vi "Get system tasklist.vi"(8 "error in (no error)":errorcluster, 11 "Task to look for":string) -> (0 "error out":errorcluster, 1 "Task found?":bool, 2 "Task count":i32, 3 "Task list":string[](array[string]))   [LabVIEW 2013]
panel:
  out "standard output":string
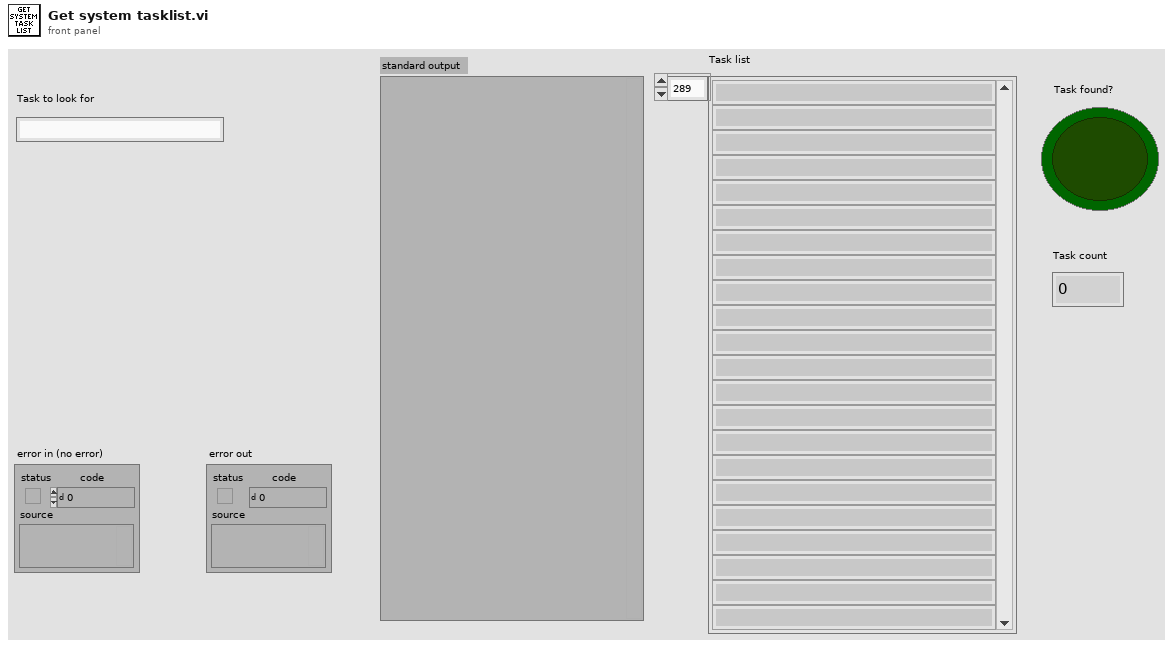
[diagram p1: front panel]
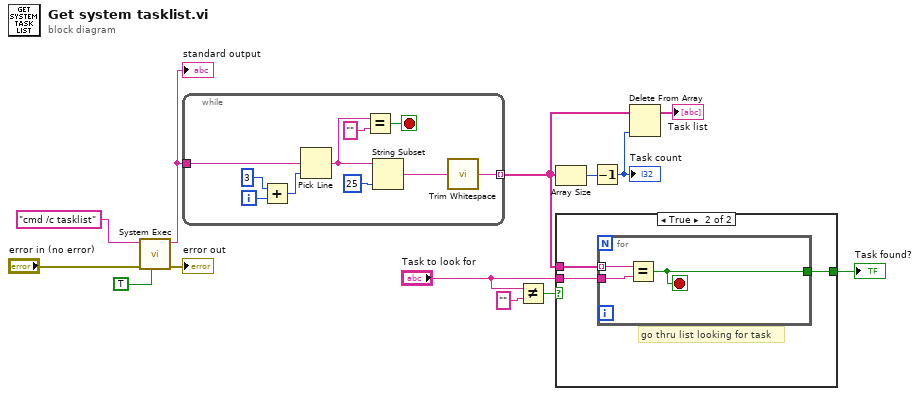
[diagram p0: block diagram]
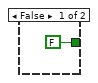
[diagram p2: hidden frame]
diagram:
  n1 = call <vilib>:"System Exec.vi"("run minimized? (F)"=TRUE, "error in (no error)"="error in (no error)", "command line"="cmd /c tasklist") -> ("error out"=→"error out":errorcluster, "standard output"=w10:string)  [unwired: 5 in, 2 out]
  "standard output" <- w10
  n2 = while {
    tunnel: w10 -> [w23]
    tunnel: [w17] -> w1 mode=indexing
    i -> [w16]
    stop <- w21 stop-if-true
    n3 = Add(x=3, y=w16) -> (x+y=w14:i32)
    n4 = Pick Line(multi-line string=w23, line index=w14) -> (output string=w20:string)  [unwired: 1 in]
    n5 = Equal?(x=w20, y="") -> (x = y?=w21:bool)
    n6 = String Subset(string=w20, length (rest)=25 ("length (rest)")) -> (substring=w18:string)  [unwired: 1 in]
    n7 = call <vilib>:"Trim Whitespace.vi"("string"=w18) -> ("trimmed string"=w17:string)  [unwired: 1 in]
  }
  n8 = Not Equal?(x="Task to look for", y="") -> (x != y?=w5:bool)
  n9 = Array Size(array=w1) -> (size(s)=w9:i32)
  n10 = case shown="True" w5 {
    tunnel: w1 -> [_ w27]
    tunnel: "Task to look for" -> [_ w26]
    tunnel: [FALSE w25] -> w3
    frame False {
    }
    frame True {
      # "go thru list looking for task"
      n11 = for {
        tunnel: w27 -> [w30] mode=indexing
        tunnel: w26 -> [w29]
        tunnel: [w28] -> w25
        stop <- w28 stop-if-true
        n12 = Equal?(x=w30, y=w29) -> (x = y?=w28:bool)
      }
    }
  }
  "Task found?" <- w3
  n13 = Decrement(x=w9) -> (x-1=w8:i32)
  "Task count" <- w8
  n14 = Delete From Array(array=w1, index=w8) -> (array with subset deleted=→"Task list":string[])  [unwired: 1 in, 1 out]
